vi "Host_AutoApproach.vi"() -> ()   [LabVIEW 2014]
uses:
  <vilib>/userdefined/High Color/nirio_resource_hc.ctl
  <vilib>/Instr/_visa.llb/VISA Configure Serial Port (Instr).vi
  <vilib>/FPGAPlugInAG/PCIe-7851R/niLvFpga_Open_PCIe-7851R.vi
  <vilib>/rvi/interface/common/dynamic/niFpgaDynamicAddResources.vi
  <vilib>/Utility/error.llb/Error Cluster From Error Code.vi
  <vilib>/rvi/errors/niLvFpgaAdjustHostInterfaceError.vi
  <vilib>/FPGAPlugInAG/Dynamic/niLvFpga_Close_Dynamic.vi
  <vilib>/rvi/interface/nirviOpenFPGA/nirviOpenFPGA.xnode
  FPGA Bitfiles/PCCrossingZProje_FPGATarget_FPGAZApproachSte_Jz78d+QsFsc.lvbitx
  <vilib>/rvi/interface/nirviReadWriteControl/nirviReadWriteControl.xnode
  <vilib>/rvi/interface/nirviCloseFPGA/nirviCloseFPGA.xnode
  FPGA Bitfiles/PCCrossingZProje_FPGATarget_FPGAZApproachSte_sDGnRDxPzNs.lvbitx
  NiFpgaLv.dll
  <vilib>/rvi/interface/Simulation/niFpgaSimulationCallBeginRW.vi
panel:
  in  "ContinuousReapproach":bool
  out "PIZRealPosDia":i16(graph)
  out "PresCurr":i16
  out "PreCurrDia":i16(graph)
  out "CalPIZPos":i16
  out "RealPIZPos":i16
  in  "stop":bool
  out "RoughZPos?":dbl
  in  "UseMemoryPos?":bool=TRUE
  in  "RoughZInitPos / mm":dbl format="%#_13g"
  out "ERR?":string
  in  "PIZ":T1
  in  "RoughZ":refnum<visa-resource-name>
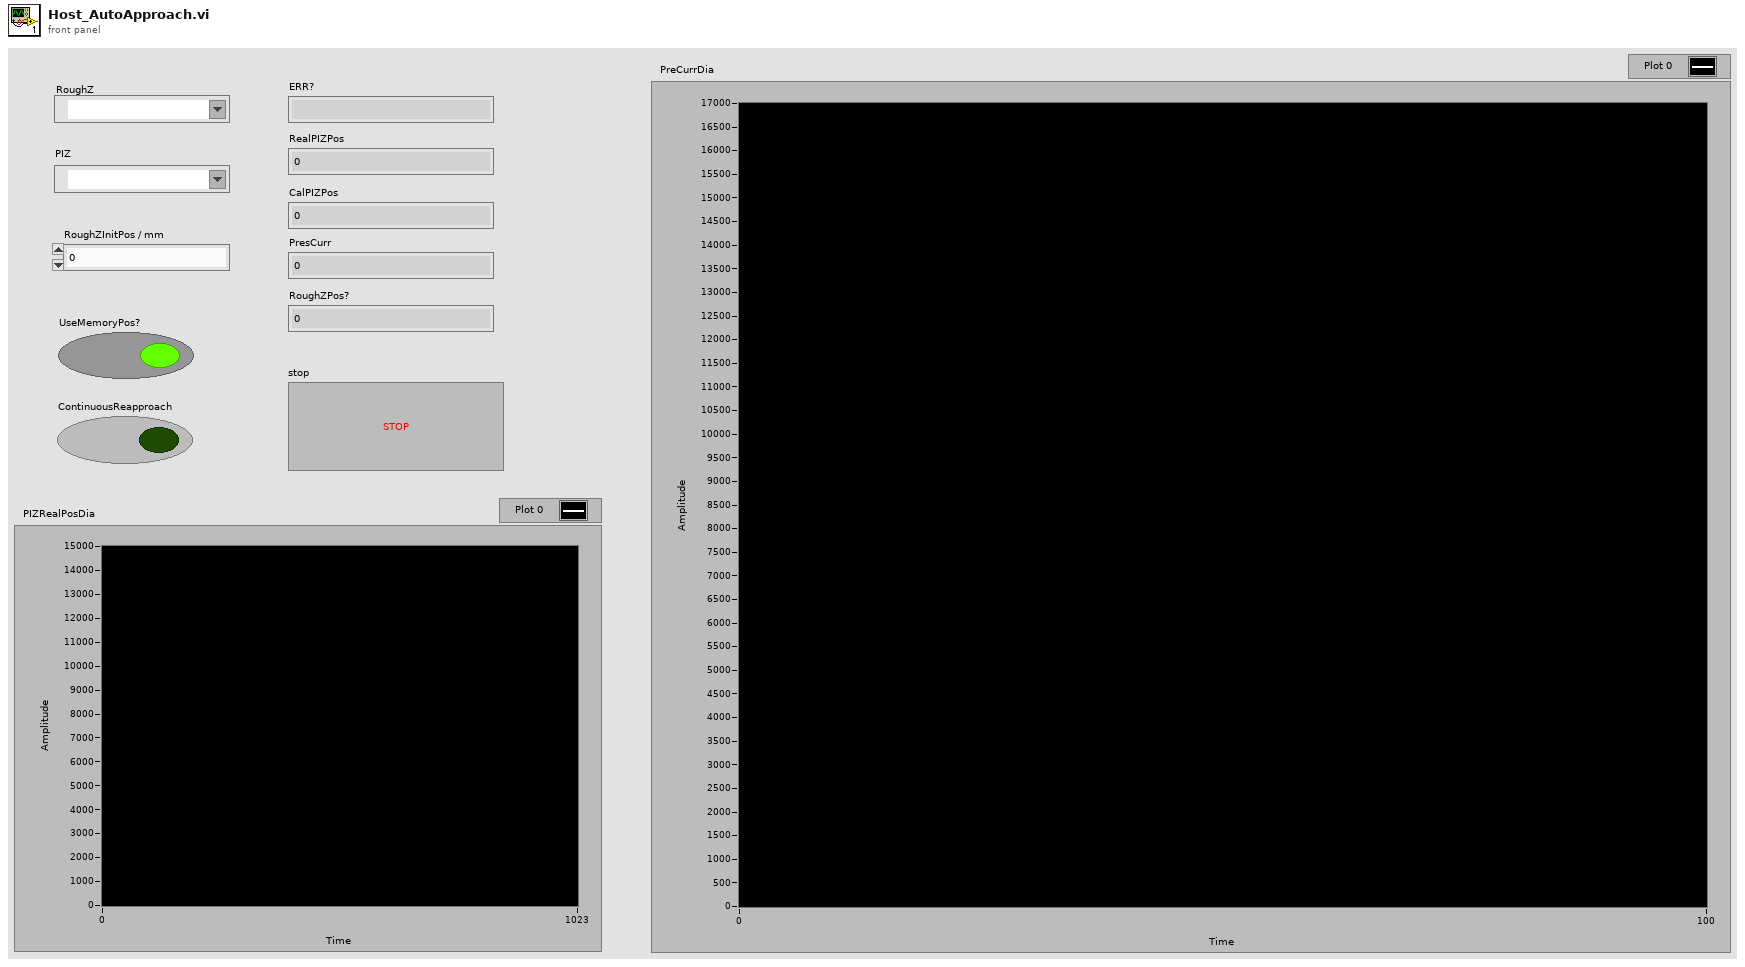
[diagram p1: front panel]
types:
  T1 = typedef "nirio_resource_hc.ctl" = tag
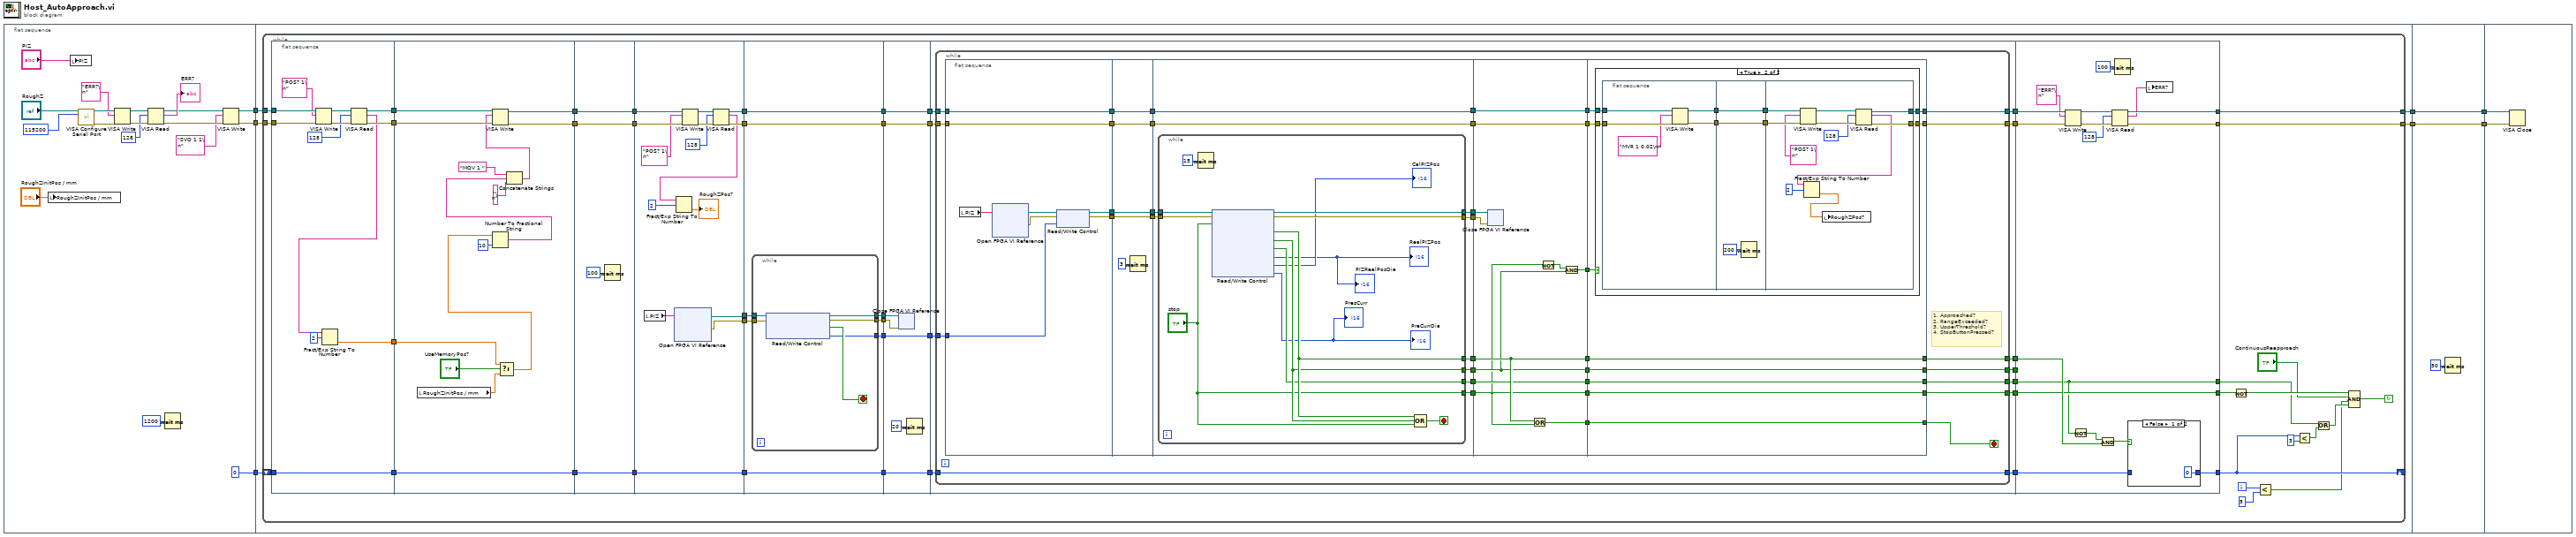
[diagram p0: block diagram]
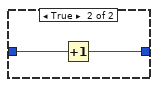
[diagram p3: hidden frame]
diagram:
  n1 = flat-sequence {
    tunnel: [w10] -> w7
    tunnel: [w9] -> w6
    tunnel: [0] -> w5
    tunnel: w7 -> [w30]
    tunnel: w6 -> [w29]
    tunnel: w5 -> [w28]
    tunnel: [w27] -> w3
    tunnel: [w26] -> w1
    tunnel: [w299] -> w4
    tunnel: w3 -> [w299]
    tunnel: [w298] -> w2
    tunnel: w1 -> [w298]
    tunnel: w4 -> [w302]
    tunnel: w2 -> [w301]
    frame #0 {
      n2 = local write "RoughZInitPos / mm"("RoughZInitPos / mm") -> ()
      n3 = local write "PIZ"("PIZ") -> ()
      n4 = call-poly "VISA Configure Serial Port"("VISA resource name"="RoughZ", "baud rate (9600)"=u32 115200) -> ("VISA resource name out"=w22:refnum<visa-resource-name>, "error out"=w21:errorcluster)  [unwired: 12 in]
      n5 = VISA Write(VISA resource name=w22, write buffer="ERR?\n", error in (no error)=w21) -> (VISA resource name out=w19:refnum<visa-resource-name>, error out=w18:errorcluster)  [unwired: 1 out]
      n6 = VISA Read(VISA resource name=w19, byte count=u32 128, error in (no error)=w18) -> (VISA resource name out=w15:refnum<visa-resource-name>, read buffer=→"ERR?":string, error out=w14:errorcluster)  [unwired: 1 out]
      n7 = Wait (ms)(milliseconds to wait=u32 1200) -> ()  [unwired: 1 out]
      n8 = VISA Write(VISA resource name=w15, write buffer="SVO 1 1\n", error in (no error)=w14) -> (VISA resource name out=w10:refnum<visa-resource-name>, error out=w9:errorcluster)  [unwired: 1 out]
    }
    frame #1 {
      n9 = while {
        tunnel: w30 -> [w79]
        tunnel: w29 -> [w78]
        shift-right: [w44] -> _
        shift-left: w28 -> [w54]
        tunnel: [w32] -> w27
        tunnel: [w31] -> w26
        i -> [w35]
        stop <- w42 continue-if-true
        n10 = flat-sequence {
          tunnel: w79 -> [w91]
          tunnel: w78 -> [w90]
          tunnel: [w85] -> w77
          tunnel: [w84] -> w76
          tunnel: [w81] -> w75
          tunnel: w54 -> [w80]
          tunnel: [w80] -> w53
          tunnel: w77 -> [w102]
          tunnel: w76 -> [w101]
          tunnel: w75 -> [w105]
          tunnel: [w94] -> w73
          tunnel: [w93] -> w71
          tunnel: w53 -> [w92]
          tunnel: [w92] -> w49
          tunnel: [w108] -> w74
          tunnel: w73 -> [w108]
          tunnel: [w107] -> w72
          tunnel: w71 -> [w107]
          tunnel: [w106] -> w50
          tunnel: w49 -> [w106]
          tunnel: w74 -> [w124]
          tunnel: w72 -> [w123]
          tunnel: [w120] -> w70
          tunnel: [w119] -> w69
          tunnel: [w112] -> w68
          tunnel: [w111] -> w67
          tunnel: [w110] -> w51
          tunnel: w50 -> [w110]
          tunnel: w70 -> [w127]
          tunnel: w69 -> [w126]
          tunnel: w68 -> [w132]
          tunnel: w67 -> [w131]
          tunnel: [w130] -> w66
          tunnel: [w129] -> w65
          tunnel: [w128] -> w64
          tunnel: [w127] -> w63
          tunnel: [w126] -> w62
          tunnel: [w125] -> w52
          tunnel: w51 -> [w125]
          tunnel: w66 -> [w142]
          tunnel: w65 -> [w141]
          tunnel: w64 -> [w140]
          tunnel: w63 -> [w144]
          tunnel: w62 -> [w143]
          tunnel: [w144] -> w61
          tunnel: [w143] -> w60
          tunnel: [w140] -> w59
          tunnel: w52 -> [w139]
          tunnel: [w139] -> w48
          tunnel: w61 -> [w156]
          tunnel: w60 -> [w155]
          tunnel: w59 -> [w154]
          tunnel: [w153] -> w58
          tunnel: [w152] -> w57
          tunnel: [w151] -> w56
          tunnel: [w150] -> w55
          tunnel: w48 -> [w149]
          tunnel: [w148] -> w47
          tunnel: [w147] -> w46
          tunnel: [w146] -> w45
          tunnel: w45 -> [w286]
          tunnel: w46 -> [w287]
          tunnel: w47 -> [w294]
          tunnel: w55 -> [w288]
          tunnel: w56 -> [w278]
          tunnel: w57 -> [_]
          tunnel: w58 -> [w291]
          tunnel: [w289] -> w44
          tunnel: [w288] -> w39
          tunnel: [w281] -> w32
          tunnel: [w280] -> w31
          tunnel: [w278] -> w36
          frame #0 {
            n11 = VISA Write(VISA resource name=w91, write buffer="POS? 1\n", error in (no error)=w90) -> (VISA resource name out=w89:refnum<visa-resource-name>, error out=w88:errorcluster)  [unwired: 1 out]
            n12 = VISA Read(VISA resource name=w89, byte count=u32 128, error in (no error)=w88) -> (VISA resource name out=w85:refnum<visa-resource-name>, read buffer=w82:string, error out=w84:errorcluster)  [unwired: 1 out]
            n13 = Fract/Exp String To Number(string=w82, offset=2) -> (number=w81:dbl)  [unwired: 2 in, 1 out]
          }
          frame #1 {
            n14 = local read "RoughZInitPos / mm"() -> (w103:dbl)
            n15 = Select(t=w105, s="UseMemoryPos?", f=w103) -> (s? t:f=w95:dbl)
            n16 = Number To Fractional String(number=w95, precision (6)=i16 10) -> (F-format string=w99:string)  [unwired: 2 in]
            n17 = Concatenate Strings("MOV 1 " ("string"), w99, "\n" ("string")) -> (w96:string)
            n18 = VISA Write(VISA resource name=w102, write buffer=w96, error in (no error)=w101) -> (VISA resource name out=w94:refnum<visa-resource-name>, error out=w93:errorcluster)  [unwired: 1 out]
          }
          frame #2 {
            n19 = Wait (ms)(milliseconds to wait=u32 100) -> ()  [unwired: 1 out]
          }
          frame #3 {
            n20 = local read "PIZ"() -> (w113:T1)
            n21 = xnode "Open FPGA VI Reference"("resource name"=w113) -> ("FPGA VI Reference Out"=w112:refnum<k20>, "error out"=w111:errorcluster)  [unwired: 1 in]
            n22 = VISA Write(VISA resource name=w124, write buffer="POS? 1\n", error in (no error)=w123) -> (VISA resource name out=w122:refnum<visa-resource-name>, error out=w121:errorcluster)  [unwired: 1 out]
            n23 = VISA Read(VISA resource name=w122, byte count=u32 128, error in (no error)=w121) -> (VISA resource name out=w120:refnum<visa-resource-name>, read buffer=w114:string, error out=w119:errorcluster)  [unwired: 1 out]
            n24 = Fract/Exp String To Number(string=w114, offset=2) -> (number=→"RoughZPos?":dbl)  [unwired: 2 in, 1 out]
          }
          frame #4 {
            n25 = while {
              tunnel: w132 -> [w138]
              tunnel: w131 -> [w137]
              tunnel: [w136] -> w130
              tunnel: [w135] -> w129
              tunnel: [w133] -> w128
              stop <- w134 stop-if-true
              n26 = xnode "Read/Write Control"("FPGA VI Reference In"=w138, "error in"=w137) -> ("FPGA VI Reference Out"=w136:refnum<k20>, "error out"=w135:errorcluster, "CurrSampleDone?"=w134:bool, "RefCurr"=w133:i16)
            }
          }
          frame #5 {
            n27 = xnode "Close FPGA VI Reference"("FPGA VI Reference In"=w142, "error in"=w141) -> ()  [unwired: 1 out]
            n28 = Wait (ms)(milliseconds to wait=u32 20) -> ()  [unwired: 1 out]
          }
          frame #6 {
            n29 = while {
              tunnel: w156 -> [w191]
              tunnel: w155 -> [w190]
              tunnel: w154 -> [w185]
              tunnel: [w163] -> w153
              tunnel: [w162] -> w152
              tunnel: [w161] -> w151
              tunnel: [w160] -> w150
              tunnel: w149 -> [w159]
              tunnel: [w159] -> w148
              tunnel: [w158] -> w147
              tunnel: [w157] -> w146
              stop <- w164 stop-if-true
              # "1. Approached?\n2. RangeExceeded?\n3. UpperThreshold?\n4. StopButtonPressed?"
              n30 = flat-sequence {
                tunnel: w191 -> [w193]
                tunnel: w190 -> [w192]
                tunnel: [w198] -> w189
                tunnel: [w195] -> w188
                tunnel: w185 -> [w194]
                tunnel: [w193] -> w184
                tunnel: [w192] -> w182
                tunnel: w189 -> [w203]
                tunnel: w188 -> [w202]
                tunnel: [w203] -> w187
                tunnel: [w202] -> w186
                tunnel: w184 -> [w201]
                tunnel: [w201] -> w183
                tunnel: w182 -> [w200]
                tunnel: [w200] -> w181
                tunnel: w187 -> [w214]
                tunnel: w186 -> [w213]
                tunnel: w183 -> [w212]
                tunnel: w181 -> [w211]
                tunnel: [w212] -> w180
                tunnel: [w211] -> w179
                tunnel: [w210] -> w178
                tunnel: [w209] -> w177
                tunnel: [w208] -> w176
                tunnel: [w207] -> w175
                tunnel: [w206] -> w174
                tunnel: [w205] -> w173
                tunnel: w180 -> [w234]
                tunnel: w179 -> [w233]
                tunnel: w178 -> [w238]
                tunnel: w177 -> [w237]
                tunnel: w176 -> [w231]
                tunnel: w175 -> [w230]
                tunnel: w174 -> [w228]
                tunnel: w173 -> [w229]
                tunnel: [w235] -> w172
                tunnel: [w234] -> w171
                tunnel: [w233] -> w170
                tunnel: [w232] -> w169
                tunnel: [w231] -> w168
                tunnel: [w230] -> w167
                tunnel: [w229] -> w166
                tunnel: [w228] -> w165
                tunnel: w172 -> [w248]
                tunnel: w171 -> [w247]
                tunnel: w170 -> [w246]
                tunnel: [w245] -> w158
                tunnel: [w244] -> w157
                tunnel: w169 -> [w239]
                tunnel: w168 -> [w243]
                tunnel: [w243] -> w163
                tunnel: w167 -> [w242]
                tunnel: [w242] -> w162
                tunnel: w166 -> [w241]
                tunnel: [w241] -> w161
                tunnel: w165 -> [w240]
                tunnel: [w240] -> w160
                tunnel: [w239] -> w164
                frame #0 {
                  n31 = local read "PIZ"() -> (w199:T1)
                  n32 = xnode "Open FPGA VI Reference"("resource name"=w199) -> ("FPGA VI Reference Out"=w197:refnum<k20>, "error out"=w196:errorcluster)  [unwired: 1 in]
                  n33 = xnode "Read/Write Control"("FPGA VI Reference In"=w197, "error in"=w196, "RefCurr"=w194) -> ("FPGA VI Reference Out"=w198:refnum<k20>, "error out"=w195:errorcluster)
                }
                frame #1 {
                  n34 = Wait (ms)(milliseconds to wait=u32 3) -> ()  [unwired: 1 out]
                }
                frame #2 {
                  n35 = while {
                    tunnel: w214 -> [w227]
                    tunnel: w213 -> [w226]
                    tunnel: [w224] -> w210
                    tunnel: [w223] -> w209
                    tunnel: [w222] -> w208
                    tunnel: [w221] -> w207
                    tunnel: ["stop"] -> w206
                    tunnel: [w219] -> w205
                    stop <- w225 stop-if-true
                    n36 = Wait (ms)(milliseconds to wait=u32 15) -> ()  [unwired: 1 out]
                    n37 = xnode "Read/Write Control"("FPGA VI Reference In"=w227, "error in"=w226, "stop"="stop") -> ("FPGA VI Reference Out"=w224:refnum<k20>, "error out"=w223:errorcluster, "Approached?"=w222:bool, "RangeExceeded?"=w221:bool, "OverUppedLimit?"=w219:bool, "RealPIZPos"=→"RealPIZPos" →"PIZRealPosDia":i16, "CalPIZPos"=→"CalPIZPos":i16, "PresCurr"=→"PreCurrDia" →"PresCurr":i16)
                    n38 = Compound Arithmetic op=OR(w222, w221, "stop") -> (w225:bool)
                  }
                }
                frame #3 {
                  n39 = xnode "Close FPGA VI Reference"("FPGA VI Reference In"=w238, "error in"=w237) -> ()  [unwired: 1 out]
                  n40 = Or(x=w231, y=w228) -> (x .or. y?=w232:bool)
                  n41 = Not(x=w228) -> (.not. x?=w236:bool)
                  n42 = And(x=w236, y=w230) -> (x .and. y?=w235:bool)
                }
                frame #4 {
                  n43 = case shown="True" w248 {
                    tunnel: w247 -> [w250 w258]
                    tunnel: w246 -> [w249 w257]
                    tunnel: [w250 w252] -> w245
                    tunnel: [w249 w251] -> w244
                    frame False {
                    }
                    frame True {
                      n44 = flat-sequence {
                        tunnel: w258 -> [w263]
                        tunnel: w257 -> [w262]
                        tunnel: [w260] -> w256
                        tunnel: [w259] -> w255
                        tunnel: w256 -> [w265]
                        tunnel: w255 -> [w264]
                        tunnel: [w265] -> w254
                        tunnel: [w264] -> w253
                        tunnel: w254 -> [w277]
                        tunnel: w253 -> [w276]
                        tunnel: [w272] -> w252
                        tunnel: [w271] -> w251
                        frame #0 {
                          n45 = VISA Write(VISA resource name=w263, write buffer="MVR 1 0.02\n", error in (no error)=w262) -> (VISA resource name out=w260:refnum<visa-resource-name>, error out=w259:errorcluster)  [unwired: 1 out]
                        }
                        frame #1 {
                          n46 = Wait (ms)(milliseconds to wait=u32 200) -> ()  [unwired: 1 out]
                        }
                        frame #2 {
                          n47 = VISA Write(VISA resource name=w277, write buffer="POS? 1\n", error in (no error)=w276) -> (VISA resource name out=w274:refnum<visa-resource-name>, error out=w273:errorcluster)  [unwired: 1 out]
                          n48 = VISA Read(VISA resource name=w274, byte count=u32 128, error in (no error)=w273) -> (VISA resource name out=w272:refnum<visa-resource-name>, read buffer=w269:string, error out=w271:errorcluster)  [unwired: 1 out]
                          n49 = Fract/Exp String To Number(string=w269, offset=2) -> (number=w267:dbl)  [unwired: 2 in, 1 out]
                          n50 = local write "RoughZPos?"(w267) -> ()
                        }
                      }
                    }
                  }
                }
              }
            }
          }
          frame #7 {
            n51 = VISA Write(VISA resource name=w287, write buffer="ERR?\n", error in (no error)=w286) -> (VISA resource name out=w284:refnum<visa-resource-name>, error out=w283:errorcluster)  [unwired: 1 out]
            n52 = Not(x=w278) -> (.not. x?=w293:bool)
            n53 = Compound Arithmetic op=AND(w293, w291) -> (w292:bool)
            n54 = VISA Read(VISA resource name=w284, byte count=u32 128, error in (no error)=w283) -> (VISA resource name out=w281:refnum<visa-resource-name>, read buffer=w279:string, error out=w280:errorcluster)  [unwired: 1 out]
            n55 = Wait (ms)(milliseconds to wait=u32 100) -> ()  [unwired: 1 out]
            n56 = case shown="False" w292 {
              tunnel: w294 -> [_ w297]
              tunnel: [0 w296] -> w289
              frame False {
              }
              frame True {
                n57 = Increment(x=w297) -> (x+1=w296:i32)
              }
            }
            n58 = local write "ERR?"(w279) -> ()
          }
        }
        n59 = Not(x=w39) -> (.not. x?=w38:bool)
        n60 = Less?(x=w35, y=5) -> (x < y?=w33:bool)
        n61 = Less?(x=w44, y=3) -> (x < y?=w41:bool)
        n62 = Or(x=w36, y=w41) -> (x .or. y?=w40:bool)
        n63 = Compound Arithmetic op=AND(w38, "ContinuousReapproach", w33, w40) -> (w42:bool)
      }
    }
    frame #2 {
      n64 = Wait (ms)(milliseconds to wait=u32 50) -> ()  [unwired: 1 out]
    }
    frame #3 {
      n65 = VISA Close(VISA resource name=w302, error in (no error)=w301) -> ()  [unwired: 1 out]
    }
  }
